vi "Library.GetTypeString.vi"(8 "error in (no error)":errorcluster, 11 "Library Reference":refnum<vi>) -> (0 "error out":errorcluster, 2 "Type String":string, 3 "Library Reference (dup)":refnum<vi>)   [LabVIEW 2011]
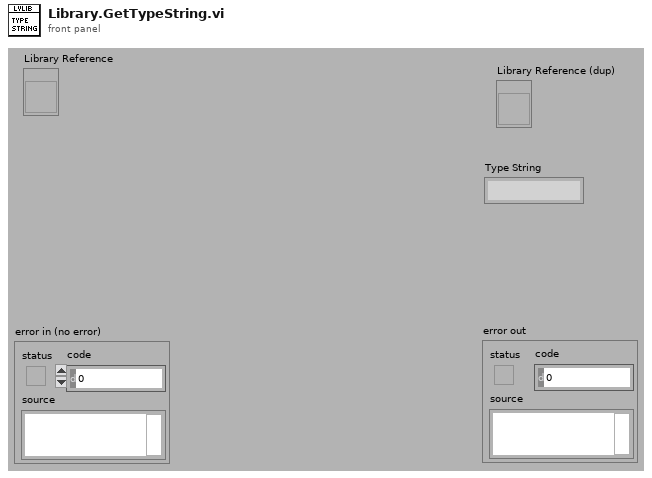
[diagram p1: front panel]
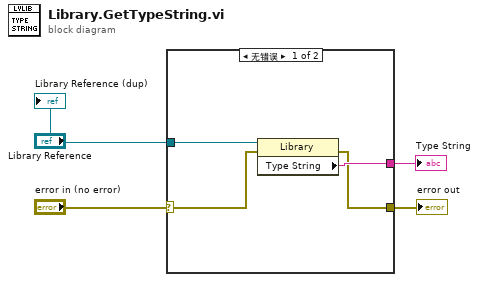
[diagram p0: block diagram]
diagram:
  n1 = case shown="无错误" "error in (no error)" {
    selector: "error in (no error)" -> [w8 w9]
    tunnel: [w7 _] -> w4
    tunnel: [w6 w9] -> w3
    tunnel: "Library Reference" -> [w5 _]
    frame No Error {
      n2 = property class="Library"(reference=w5, error in=w8) -> (error out=w6:errorcluster, "Type String"=w7:string)  [unwired: 1 out]
    }
    frame Error {
    }
  }
  "Type String" <- w4
  "error out" <- w3
  "Library Reference (dup)" <- "Library Reference"
